vi "Decompose VI (Refnum).vi"(8 "error in (no error)":errorcluster, 11 "VI Ref":refnum<vi>) -> (0 "error out":errorcluster, 1 "Block Diagram XML":string, 2 "Front Panel XML":string, 3 "VI Ref out":refnum<vi>, 4 "Other resources":T1[](array[typedef]))   [LabVIEW 2026, in "VILab.lvlib"]
uses:
  VILab.lvlib
  CTLs/Resource.ctl
  <vilib>/Utility/error.llb/Error Cluster From Error Code.vi
  Find Resource by Type (String).vi
  <vilib>/ErrorRing/Error Ring.xnode
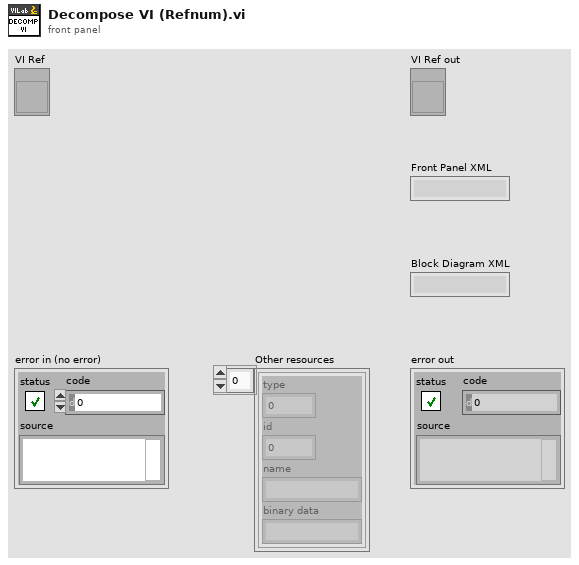
[diagram p1: front panel]
types:
  T1 = typedef "VILab.lvlib/Resource.ctl" = cluster{"type":u32, "id":i32, "name":string, "binary data":string}
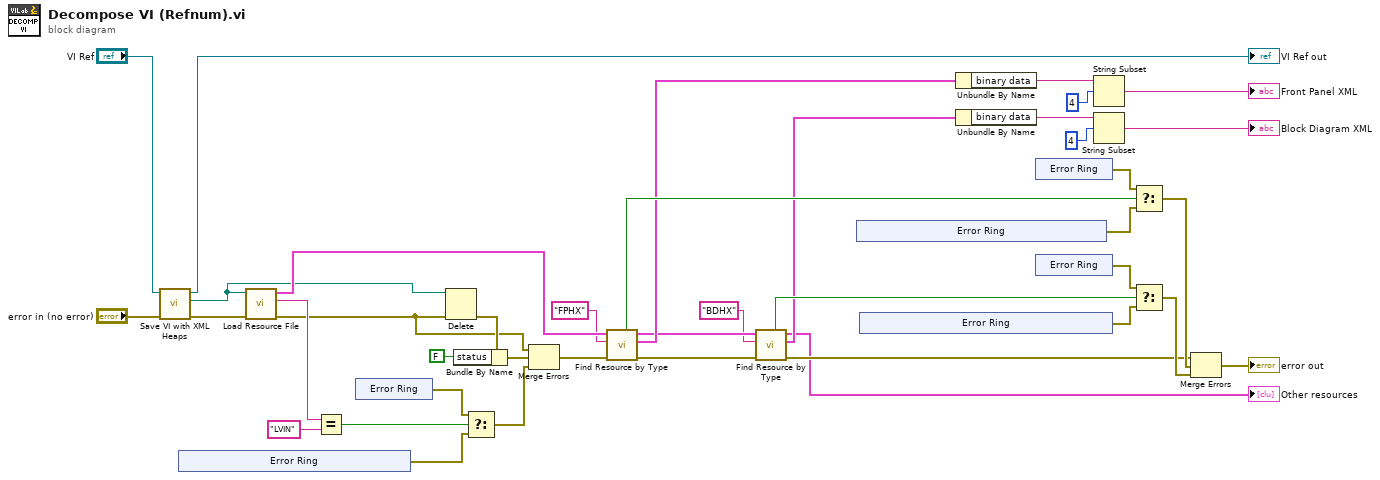
[diagram p0: block diagram]
diagram:
  n1 = call "Save VI with XML Heaps.vi"("error in (no error)"="error in (no error)", "VI Refnum In"="VI Ref") -> ("error out"=w39:errorcluster, "VI Path out"=w16:path, "VI Refnum Out"=→"VI Ref out":refnum<vi>)  [unwired: 7 in]
  n2 = xnode "Error Ring"() -> ("error out"=w33:errorcluster)
  n3 = call "Load Resource File.vi"("error in (no error)"=w39, "Resource File"=w16) -> ("error out"=w20:errorcluster, "File Type"=w36:string, "Resources"=w31:T1[])  [unwired: 7 in]
  n4 = Equal?(x=w36, y="LVIN") -> (x = y?=w34:bool)
  n5 = xnode "Error Ring"() -> ("error out"=w1:errorcluster)
  n6 = Delete(path (use dialog)=w16, error in=w20) -> (error out=w38:errorcluster)  [unwired: 3 in, 2 out]
  n7 = Bundle By Name(cluster=w38, "status"=FALSE) -> (w21:errorcluster)
  n8 = Select(t=w1, s=w34, f=w33) -> (s? t:f=w32:errorcluster)
  n9 = Merge Errors(w20, w21, w32) -> (w25:errorcluster)
  n10 = call-poly "Find Resource by Type.vi"("error in (no error)"=w25, "Resource Type"="FPHX", "Resources"=w31) -> ("error out"=w4:errorcluster, "Resource"=w12:T1, "Resources out"=w10:T1[], "Found?"=w14:bool)  [unwired: 4 in, 1 out]
  n11 = call-poly "Find Resource by Type.vi"("error in (no error)"=w4, "Resource Type"="BDHX", "Resources"=w10) -> ("error out"=w19:errorcluster, "Resource"=w11:T1, "Resources out"=→"Other resources":T1[], "Found?"=w13:bool)  [unwired: 4 in, 1 out]
  n12 = xnode "Error Ring"() -> ("error out"=w3:errorcluster)
  n13 = xnode "Error Ring"() -> ("error out"=w7:errorcluster)
  n14 = Unbundle By Name(w12) -> ("binary data"=w30:string)
  n15 = Unbundle By Name(w11) -> ("binary data"=w29:string)
  n16 = xnode "Error Ring"() -> ("error out"=w5:errorcluster)
  n17 = xnode "Error Ring"() -> ("error out"=w6:errorcluster)
  n18 = String Subset(string=w30, offset (0)=4) -> (substring=→"Front Panel XML":string)  [unwired: 1 in]
  n19 = String Subset(string=w29, offset (0)=4) -> (substring=→"Block Diagram XML":string)  [unwired: 1 in]
  n20 = Select(t=w5, s=w14, f=w3) -> (s? t:f=w23:errorcluster)
  n21 = Select(t=w6, s=w13, f=w7) -> (s? t:f=w24:errorcluster)
  n22 = Merge Errors(w19, w23, w24) -> (→"error out":errorcluster)
